vi "SpreadsheetRead.vi"() -> ()   [LabVIEW 2015]
uses:
  <vilib>/Utility/file.llb/Read Delimited Spreadsheet (DBL).vi
panel:
  out "output cluster":cluster{"all rows":dbl[], "all rows":dbl[]}
  out "XY Graph":cluster{"all rows":dbl[], "all rows":dbl[]}(graph)
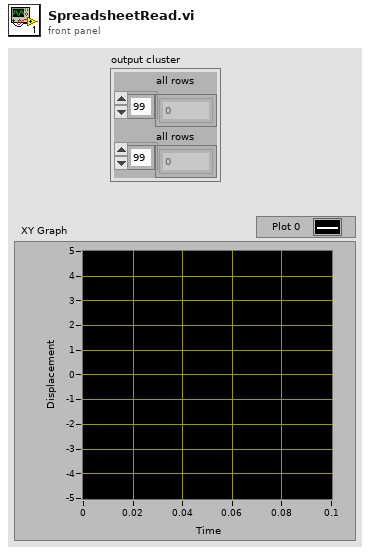
[diagram p1: front panel]
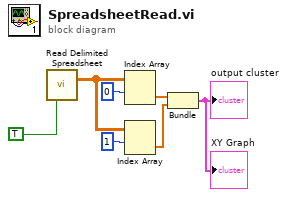
[diagram p0: block diagram]
diagram:
  n1 = call-poly <vilib>:"Read Delimited Spreadsheet.vi"("transpose? (F)"=TRUE) -> ("all rows"=w5:dbl[][])  [unwired: 9 in, 5 out]
  n2 = Index Array(array=w5, index (row)=0) -> (element=w3:dbl[])  [unwired: 1 in]
  n3 = Index Array(array=w5, index (row)=1) -> (element=w4:dbl[])  [unwired: 1 in]
  n4 = Bundle("all rows"=w3, "all rows"=w4) -> (→"XY Graph" →"output cluster":cluster{"all rows":dbl[], "all rows":dbl[]})  [unwired: 1 in]
